vi "TCL Init.vi"(0 "config file":path, 5 "error in (no error)":errorcluster) -> (14 "event file":path, 16 "fragments":string[](array[string]), 17 "signals":string[](array[string]), 18 "primary key":string, 19 "error out":errorcluster)   [LabVIEW 2010]
uses:
  <vilib>/Utility/config.llb/Read Key (String).vi
  TCL Global.vi
  <vilib>/Utility/config.llb/NI_LVConfig.lvlib
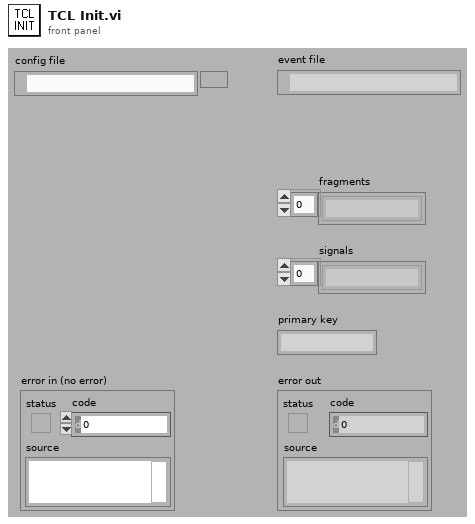
[diagram p1: front panel]
types:
  T1 = typedef "NI_LVConfig.lvlib/Config Data RefNum.ctl" = refnum<k1>
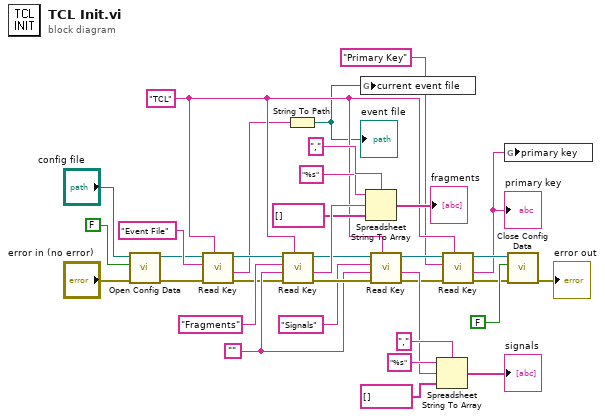
[diagram p0: block diagram]
diagram:
  w17 = ""
  w9 = "TCL" ("section")
  n1 = call <vilib>:"Open Config Data.vi"("error in (no error)"="error in (no error)", "create file if necessary (T)"=FALSE, "configuration file path"="config file") -> ("error out"=w3:errorcluster, "refnum"=w2:T1)  [unwired: 6 in, 1 out]
  n2 = call-poly <vilib>:"Read Key.vi"("section"=w9, "error in (no error)"=w3, "key"="Event File", "refnum"=w2) -> ("error out"=w14:errorcluster, "value"=w5:string, "refnum out"=w13:T1)  [unwired: 4 in, 1 out]
  n3 = call-poly <vilib>:"Read Key.vi"("section"=w9, "error in (no error)"=w14, "default value"=w17, "key"="Fragments", "refnum"=w13) -> ("error out"=w18:errorcluster, "value"=w29:string, "refnum out"=w19:T1)  [unwired: 3 in, 1 out]
  n4 = String To Path(string=w5) -> (path=w1:path)
  "event file" <- w1
  n5 = global write "TCL Global.vi" "current event file"(w1) -> ()
  n6 = Spreadsheet String To Array(delimiter (Tab)=",", format string="%s", spreadsheet string=w29, array type (2D Dbl)=string[] []) -> (array=→"fragments":string[])
  n7 = call-poly <vilib>:"Read Key.vi"("section"=w9, "error in (no error)"=w18, "default value"=w17, "key"="Signals", "refnum"=w19) -> ("error out"=w10:errorcluster, "value"=w15:string, "refnum out"=w11:T1)  [unwired: 3 in, 1 out]
  n8 = Spreadsheet String To Array(delimiter (Tab)=",", format string="%s", spreadsheet string=w15, array type (2D Dbl)=string[] []) -> (array=→"signals":string[])
  n9 = call-poly <vilib>:"Read Key.vi"("section"=w9, "error in (no error)"=w10, "key"="Primary Key", "refnum"=w11) -> ("error out"=w6:errorcluster, "value"=w4:string, "refnum out"=w7:T1)  [unwired: 4 in, 1 out]
  "primary key" <- w4
  n10 = global write "TCL Global.vi" "primary key"(w4) -> ()
  n11 = call <vilib>:"Close Config Data.vi"("error in (no error)"=w6, "write file if changed (T)"=FALSE, "refnum"=w7) -> ("error out"=→"error out":errorcluster)  [unwired: 7 in, 1 out]
